vi "十六进制转ASCII字符串多态.vi"   [LabVIEW 2016, in "环境动力监测库.lvlib" / "空调库.lvlib"]
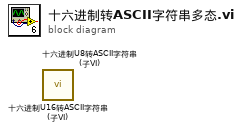
[diagram p0: block diagram]
diagram:
  n1 = call "十六进制U16转ASCII字符串 (子VI).vi"() -> ()  [unwired: 11 in, 1 out]
  n2 = call "十六进制U8转ASCII字符串 (子VI).vi"() -> ()  [unwired: 11 in, 1 out]
